vi "FPGA_myRIO_19500_camera_trigger.vi"() -> ()   [LabVIEW 2019]
doc: "The myRIO v1.1 FPGA Shipping Personality. This personality contains support for:\n- 2 Analog Input Interrupt channel\n- 4 Digital Input Interrupt channel\n- 1 Timer\n- 1 Accelerometer\n- 1 Button\n- 4 LED\n- 10 Analog Input channels with 1 Sample\n- 6 Analog Output channels with 1 Sample\n- 40 Digital I/O channels with 1 Sample\n- 2 I2C channels\n- 4 Encoder channels\n- 6 PWM channels\n- 2 SPI channels"
uses:
  <vilib>/rvi/Emulation/niFpgaGetClockAttributes.vi
  <vilib>/rvi/Emulation/niFpgaSctlEmulationGetInTimedLoop.vi
  <vilib>/rvi/Emulation/niFpgaEmulationReportErrorSimple.vi
  <vilib>/rvi/Emulation/niFpgaProcessEmulError.vi
  <vilib>/rvi/Emulation/niFpgaCriticalErrorInLSC.vi
  <vilib>/rvi/eio/common/nirviEmuTemplateMethod_errors.vi
  <vilib>/eio/EIONode/EIONode.xnode
panel:
  out "PinMap":bool[](array[boolean])
  in  "SequenceSIze":u64
  in  "PinArray":u8[](array[numeric])=[0, 0, 0, 0, 0, 0, 0, 0]
  out "LoopNumber":u64
  in  "OutputPinMap":u8
  in  "Sequence":bool
  out "PulseNumber":u64
  in  "Synchronization":bool
  out "DIO_indicator":bool[](array[boolean])
  out "Camera_triggerin":bool
  out "Camera_triggerout":bool
  in  "PulseNumberperLoop":i32
  in  "Trigger":u64
  in  "BreakinLoop":bool
  in  "OFFTime":u32
  in  "ONTime":u32
  # "Camera trigger port: A:DIO8\nCamera trigger in port A:DIO15\nLight source port: B:DIO1~7, 1~6 are Normally Open (NO), 7 is  NC."
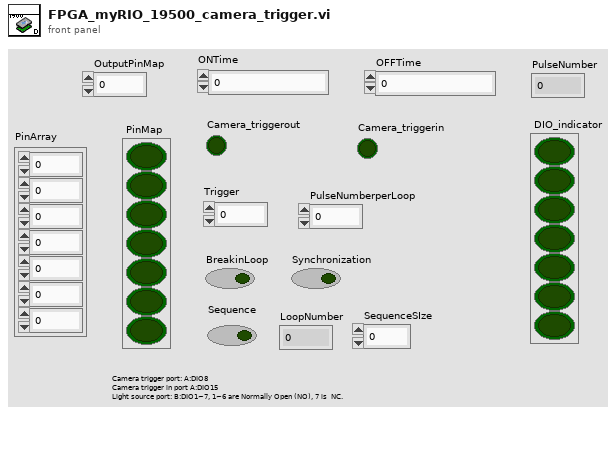
[diagram p1: front panel]
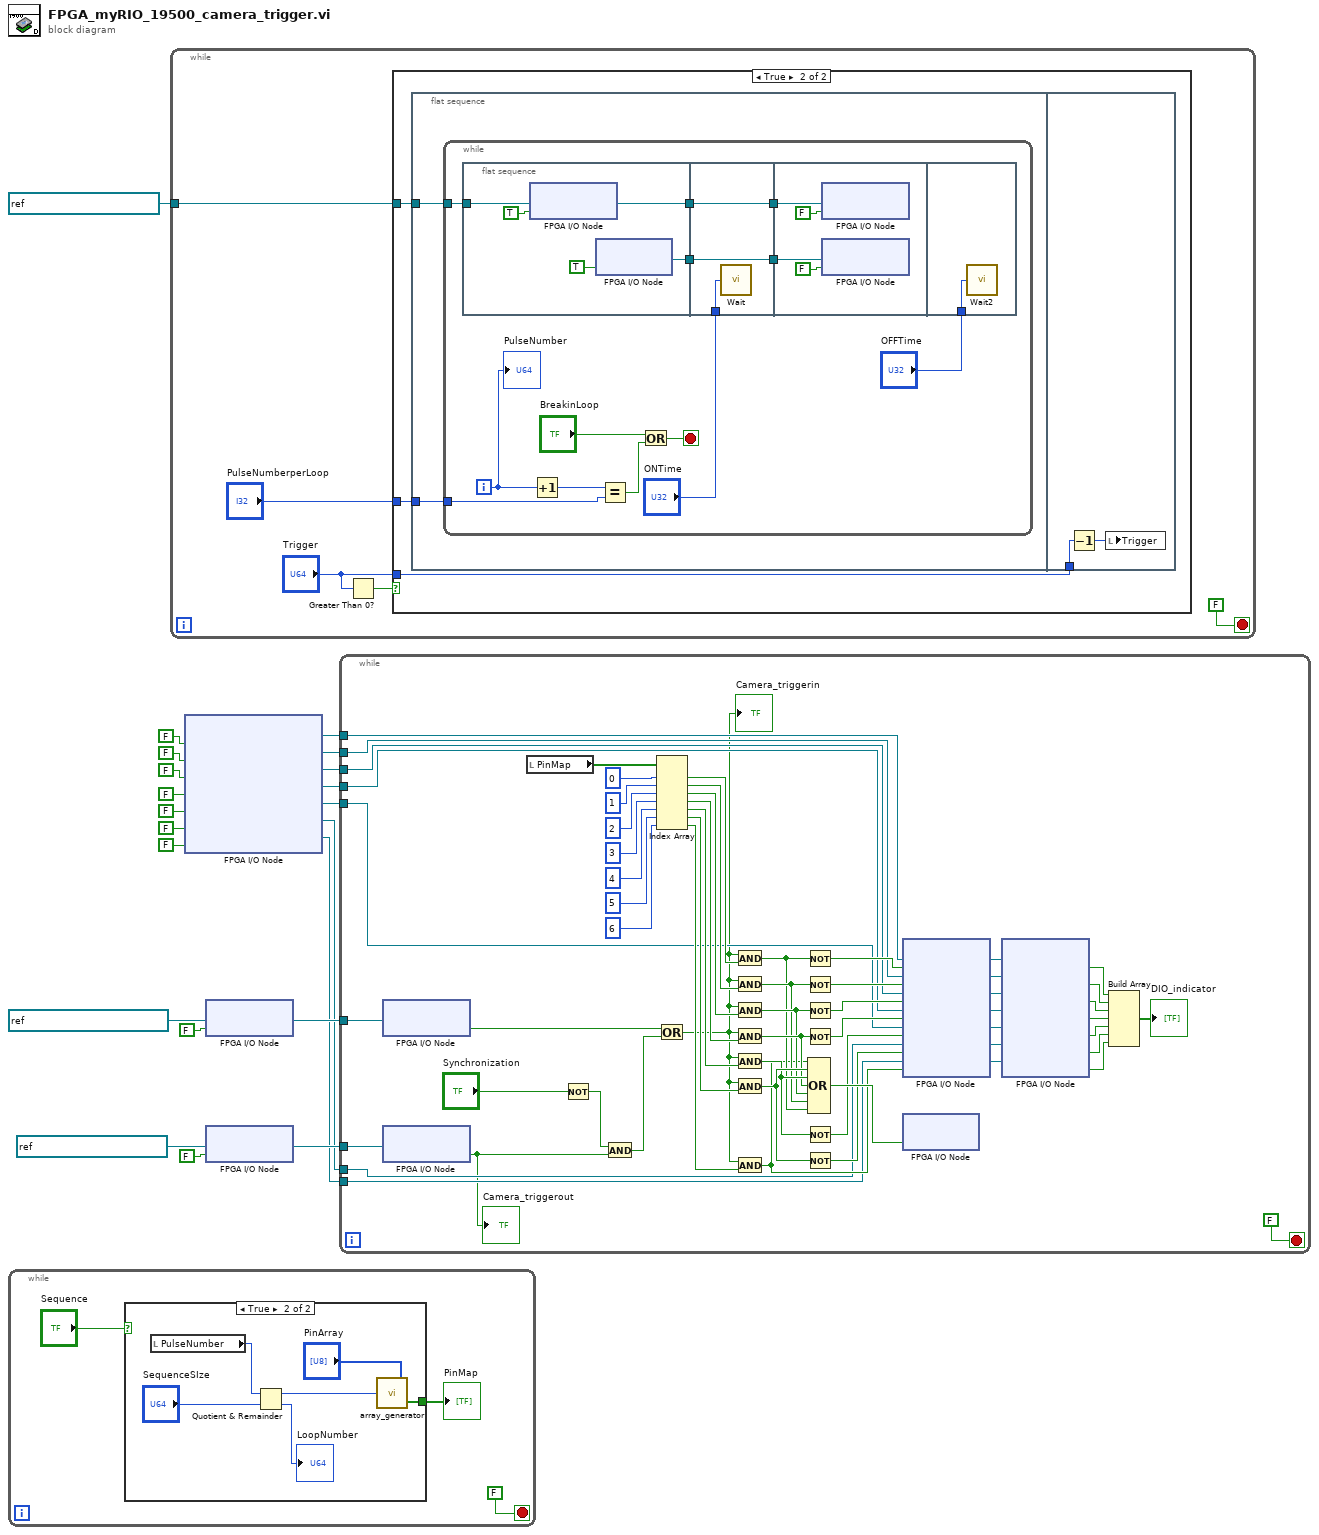
[diagram p0: block diagram]
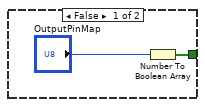
[diagram p2: hidden frame]
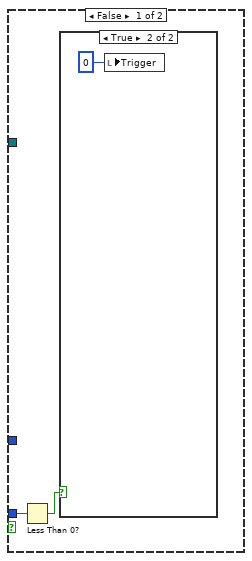
[diagram p3: hidden frame]
diagram:
  n1 = while {
    stop <- FALSE stop-if-true
    n2 = case shown="True" "Sequence" {
      tunnel: [w25 w30] -> w23
      frame False {
        n3 = Number To Boolean Array(number="OutputPinMap") -> (Boolean array=w25:bool[])
      }
      frame True {
        n4 = local read "PulseNumber"() -> (w27:u64)
        n5 = Quotient & Remainder(x=w27, y="SequenceSIze") -> (x-y*floor(x/y)=w31:u64, floor(x/y)=→"LoopNumber":u64)
        n6 = call "array_generator.vi"("Index"=w31, "Array"="PinArray") -> ("Boolean array"=w30:bool[])
      }
    }
    "PinMap" <- w23
  }
  n7 = while {
    tunnel: refnum<k21> "ConnectorA/DIO8" ("FPGA I/O In") -> [w33]
    stop <- FALSE stop-if-true
    n8 = Greater Than 0?(x="Trigger") -> (x > 0?=w36:bool)
    n9 = case shown="True" w36 {
      tunnel: "PulseNumberperLoop" -> [_ w43]
      tunnel: "Trigger" -> [w39 w42]
      tunnel: w33 -> [_ w41]
      frame False {
        n10 = Less Than 0?(x=w39) -> (x < 0?=w38:bool)
        n11 = case shown="True" w38 {
          frame False {
          }
          frame True {
            n12 = local write "Trigger"(i16 0) -> ()
          }
        }
      }
      frame True {
        n13 = flat-sequence {
          tunnel: w43 -> [w45]
          tunnel: w41 -> [w44]
          tunnel: w42 -> [w72]
          frame #0 {
            n14 = while {
              tunnel: w45 -> [w54]
              tunnel: w44 -> [w46]
              i -> [w47]
              stop <- w56 stop-if-true
              n15 = flat-sequence {
                tunnel: [w61] -> w50
                tunnel: [w60] -> w48
                tunnel: w46 -> [w59]
                tunnel: "ONTime" -> [w66]
                tunnel: [w65] -> w51
                tunnel: w50 -> [w65]
                tunnel: [w64] -> w49
                tunnel: w48 -> [w64]
                tunnel: w51 -> [w68]
                tunnel: w49 -> [w67]
                tunnel: "OFFTime" -> [w71]
                frame #0 {
                  n16 = xnode "FPGA I/O Node"("I/O Item"=TRUE ("ConnectorA/DIO8"), "FPGA I/O In"=w59) -> ("FPGA I/O Out"=w60:refnum<k21>)
                  n17 = xnode "FPGA I/O Node"("LED0"=TRUE ("ConnectorA/DIO8")) -> ("FPGA I/O Out"=w61:refnum<k21>)  [unwired: 1 in]
                }
                frame #1 {
                  n18 = call "Wait"("Count(uSec)"=w66) -> ()  [unwired: 1 out]
                }
                frame #2 {
                  n19 = xnode "FPGA I/O Node"("I/O Item"=FALSE ("ConnectorA/DIO8"), "FPGA I/O In"=w67) -> ()  [unwired: 1 out]
                  n20 = xnode "FPGA I/O Node"("I/O Item"=FALSE ("ConnectorA/DIO8"), "FPGA I/O In"=w68) -> ()  [unwired: 1 out]
                }
                frame #3 {
                  n21 = call "Wait2"("Count(uSec)"=w71) -> ()  [unwired: 1 out]
                }
              }
              n22 = Increment(x=w47) -> (x+1=w55:i32)
              n23 = Equal?(x=w55, y=w54) -> (x = y?=w58:bool)
              n24 = Or(x="BreakinLoop", y=w58) -> (x .or. y?=w56:bool)
              "PulseNumber" <- w47
            }
          }
          frame #1 {
            n25 = Decrement(x=w72) -> (x-1=w73:u64)
            n26 = local write "Trigger"(w73) -> ()
          }
        }
      }
    }
  }
  n27 = xnode "FPGA I/O Node"("ConnectorB/DIO1"=FALSE ("ConnectorC/DIO1"), "ConnectorB/DIO2"=FALSE ("ConnectorC/DIO2"), "ConnectorB/DIO3"=FALSE ("ConnectorC/DIO3"), "ConnectorB/DIO4"=FALSE ("ConnectorC/DIO4"), "ConnectorB/DIO5"=FALSE ("ConnectorC/DIO5"), "ConnectorB/DIO6"=FALSE ("ConnectorC/DIO6"), "ConnectorB/DIO7"=FALSE ("ConnectorC/DIO7")) -> ("FPGA I/O Out"=w8:refnum<k21>, "FPGA I/O Out"=w7:refnum<k21>, "FPGA I/O Out"=w6:refnum<k21>, "FPGA I/O Out"=w5:refnum<k21>, "FPGA I/O Out"=w4:refnum<k21>, "FPGA I/O Out"=w3:refnum<k21>, "FPGA I/O Out"=w2:refnum<k21>)  [unwired: 7 in]
  n28 = xnode "FPGA I/O Node"("I/O Item"=FALSE ("ConnectorB/DIO7"), "FPGA I/O In"=refnum<k21> "ConnectorA/DIO15") -> ("FPGA I/O Out"=w15:refnum<k21>)
  n29 = xnode "FPGA I/O Node"("I/O Item"=FALSE ("ConnectorA/DIO8"), "FPGA I/O In"=refnum<k21> "ConnectorA/DIO8") -> ("FPGA I/O Out"=w18:refnum<k21>)
  n30 = while {
    tunnel: w18 -> [w96]
    tunnel: w15 -> [w95]
    tunnel: w8 -> [w94]
    tunnel: w7 -> [w93]
    tunnel: w6 -> [w92]
    tunnel: w5 -> [w91]
    tunnel: w4 -> [w90]
    tunnel: w3 -> [w89]
    tunnel: w2 -> [w88]
    stop <- FALSE stop-if-true
    n31 = xnode "FPGA I/O Node"("FPGA I/O In"=w95) -> ("I/O Item"=w85:bool)  [unwired: 1 out]
    n32 = xnode "FPGA I/O Node"("FPGA I/O In"=w96) -> ("I/O Item"=w75:bool)  [unwired: 1 out]
    "Camera_triggerout" <- w75
    n33 = local read "PinMap"() -> (w74:bool[])
    n34 = Not(x="Synchronization") -> (.not. x?=w83:bool)
    n35 = And(x=w83, y=w75) -> (x .and. y?=w84:bool)
    n36 = Index Array(array=w74, index #1=0 ("index"), index #2=1 ("index"), index #3=2 ("index"), index #4=3 ("index"), index #5=4 ("index"), index #6=5 ("index"), index #7=6 ("index")) -> (element #1=w122:bool, element #2=w121:bool, element #3=w120:bool, element #4=w119:bool, element #5=w118:bool, element #6=w117:bool, element #7=w116:bool)
    n37 = Or(x=w85, y=w84) -> (x .or. y?=w86:bool)
    "Camera_triggerin" <- w86
    n38 = And(x=w86, y=w122) -> (x .and. y?=w110:bool)
    n39 = And(x=w86, y=w121) -> (x .and. y?=w111:bool)
    n40 = And(x=w86, y=w120) -> (x .and. y?=w112:bool)
    n41 = And(x=w86, y=w119) -> (x .and. y?=w113:bool)
    n42 = And(x=w86, y=w118) -> (x .and. y?=w114:bool)
    n43 = And(x=w86, y=w117) -> (x .and. y?=w115:bool)
    n44 = And(x=w86, y=w116) -> (x .and. y?=w104:bool)
    n45 = Not(x=w110) -> (.not. x?=w123:bool)
    n46 = Not(x=w111) -> (.not. x?=w124:bool)
    n47 = Not(x=w112) -> (.not. x?=w108:bool)
    n48 = Not(x=w113) -> (.not. x?=w107:bool)
    n49 = Not(x=w114) -> (.not. x?=w106:bool)
    n50 = Not(x=w115) -> (.not. x?=w105:bool)
    n51 = Compound Arithmetic op=OR(w104, w115, w114, w113, w112, w111, w110) -> (w109:bool)
    n52 = xnode "FPGA I/O Node"("I/O Item"=w123, "FPGA I/O In"=w94, "I/O Item"=w124, "FPGA I/O In"=w93, "I/O Item"=w108, "FPGA I/O In"=w92, "I/O Item"=w107, "FPGA I/O In"=w91, "I/O Item"=w106, "FPGA I/O In"=w90, "I/O Item"=w105, "FPGA I/O In"=w89, "I/O Item"=w104, "FPGA I/O In"=w88) -> ("FPGA I/O Out"=w103:refnum<k21>, "FPGA I/O Out"=w102:refnum<k21>, "FPGA I/O Out"=w101:refnum<k21>, "FPGA I/O Out"=w100:refnum<k21>, "FPGA I/O Out"=w99:refnum<k21>, "FPGA I/O Out"=w98:refnum<k21>, "FPGA I/O Out"=w97:refnum<k21>)
    n53 = xnode "FPGA I/O Node"("LED1"=w109) -> ()  [unwired: 1 in, 1 out]
    n54 = xnode "FPGA I/O Node"("FPGA I/O In"=w103, "FPGA I/O In"=w102, "FPGA I/O In"=w101, "FPGA I/O In"=w100, "FPGA I/O In"=w99, "FPGA I/O In"=w98, "FPGA I/O In"=w97) -> ("I/O Item"=w125:bool, "I/O Item"=w126:bool, "I/O Item"=w127:bool, "I/O Item"=w128:bool, "I/O Item"=w129:bool, "I/O Item"=w130:bool, "I/O Item"=w131:bool)  [unwired: 7 out]
    n55 = Build Array(w125, w126, w127, w128, w129, w130, w131) -> (→"DIO_indicator":bool[])
  }
